vi "Configure Timing.vi"(8 "error in":errorcluster, 11 "DAQmx Base Configure Strategy in":refnum<class "DAQmx Base Configure Strategy.lvclass">) -> (0 "error out":errorcluster, 3 "DAQmx Base Configure Strategy out":refnum<class "DAQmx Base Configure Strategy.lvclass">)   [LabVIEW 2024, in "DAQmx Base Configure Strategy.lvclass"]
uses:
  DAQmx Base Configure Strategy.lvclass
  DAQmx Base Configure Strategy.lvclass/DAQmx Base Configure Strategy.ctl
  65035ada-ba25-4b4b-831a-509cfaf4f843.vi
  Source/Interfaces/IConfiguration/IConfiguration.lvclass
  <vilib>/DAQmx/configure/timing.llb/DAQmx Timing (Sample Clock).vi
  <vilib>/DAQmx/configure/timing.llb/DAQmx Timing (Implicit).vi
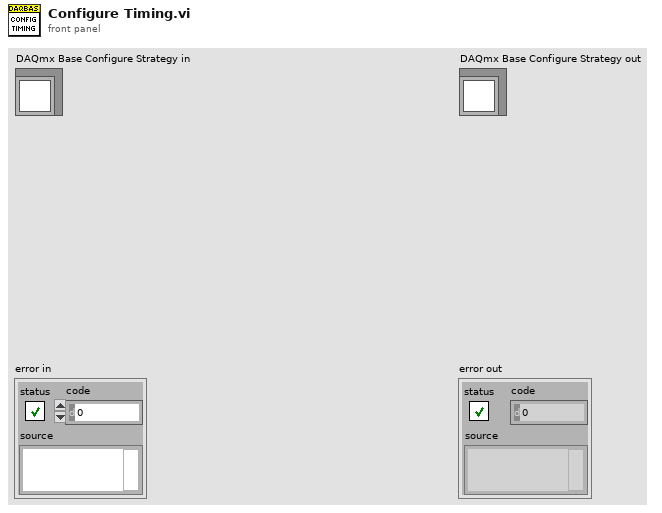
[diagram p1: front panel]
types:
  T1 = cluster{"Type":string, "SamplesPerChannel":i32, "SampleMode":string, "SampleRate":dbl, "SampleClockSource":string, "ActiveEdge":string}
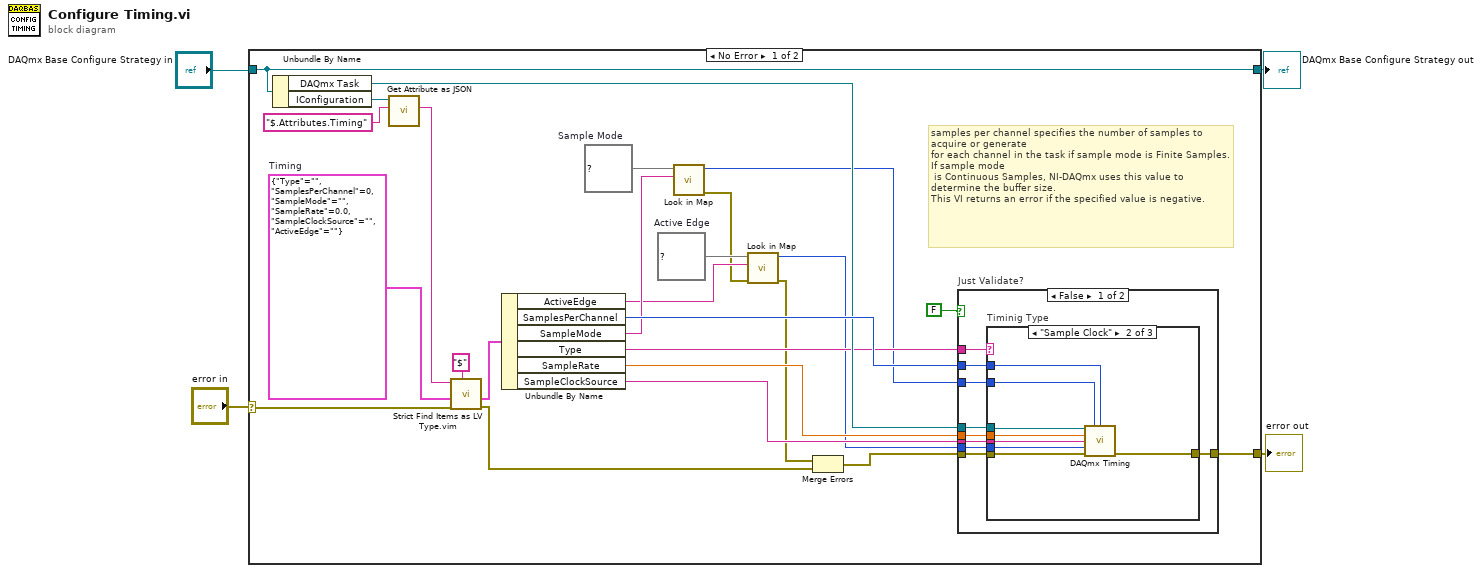
[diagram p0: block diagram]
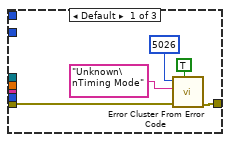
[diagram p2: hidden frame]
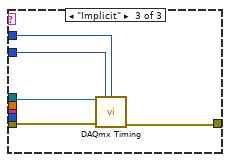
[diagram p3: hidden frame]
diagram:
  n1 = case shown="No Error" "error in" {
    selector: "error in" -> [w20 w59]
    tunnel: [w23 w59] -> w1
    tunnel: "DAQmx Base Configure Strategy in" -> [w13 w58]
    tunnel: [w13 w58] -> w3
    frame No Error {
      w16 = map{string, i32} {"Falling"=10171, "Rising"=10280}  # Active Edge
      w19 = map{string, i32} {"Continuous Samples"=10123, "Finite Samples"=10178, "Hardware Timed Single Point"=12522}  # Sample Mode
      w29 = T1 {"Type"="", "SamplesPerChannel"=0, "SampleMode"="", "SampleRate"=0.0, "SampleClockSource"="", "ActiveEdge"=""}  # Timing
      # "samples per channel specifies the number of samples to acquire or generate\nfor each channel in the task if sample mode is Finite Samples. If sample mode\n is Continuous Samples, NI-DAQmx uses this value to determine the buffer size.\nThis VI returns an error if the specified value is negative."
      n2 = Unbundle By Name(w13) -> ("DAQmx Task"=w24:refnum<k21>, "IConfiguration"=w8:refnum<class "IConfiguration.lvclass">)
      n3 = call-dynamic "Get Attribute as JSON.vi"("Attribute"="$.Attributes.Timing", "IConfiguration in"=w8) -> ("<JSON>"=w11:string)  [unwired: 7 in, 2 out]
      n4 = call "Strict Find Items as LV Type.vim"("$Path or Item Name"="$", "error in"=w20, "Data Type and Default Value"=w29, "<JSON>"=w11) -> ("error out"=w5:errorcluster, "Data out"=w28:T1)  [unwired: 5 in, 1 out]
      n5 = Unbundle By Name(w28) -> ("ActiveEdge"=w15:string, "SamplesPerChannel"=w25:i32, "SampleMode"=w18:string, "Type"=w22:string, "SampleRate"=w26:dbl, "SampleClockSource"=w27:string)
      n6 = call "Look in Map.vi"("key"=w18, "map"=w19) -> ("error out"=w7:errorcluster, "value"=w17:i32)  [unwired: 8 in]
      n7 = call "Look in Map.vi"("error in"=w7, "key"=w15, "map"=w16) -> ("error out"=w6:errorcluster, "value"=w14:i32)  [unwired: 7 in]
      n8 = Merge Errors(w6, w5) -> (w21:errorcluster)
      n9 = case "Just Validate?" shown="False" FALSE {
        tunnel: w21 -> [w38 w57]
        tunnel: w27 -> [w37 _]
        tunnel: w26 -> [w36 _]
        tunnel: w17 -> [w35 _]
        tunnel: w25 -> [w34 _]
        tunnel: w24 -> [w33 _]
        tunnel: w14 -> [w32 _]
        tunnel: [w31 w57] -> w23
        tunnel: w22 -> [w30 _]
        frame False {
          n10 = case "Timinig Type" shown="\"Sample Clock\"" w30 {
            tunnel: w38 -> [w42 w51 w54]
            tunnel: w37 -> [_ w50 _]
            tunnel: w36 -> [_ w49 _]
            tunnel: w35 -> [_ w48 w53]
            tunnel: w34 -> [_ w47 w52]
            tunnel: w33 -> [_ w46 w55]
            tunnel: [w43 w45 w56] -> w31
            tunnel: w32 -> [_ w44 _]
            frame Default {
              n11 = call <vilib>:"Error Cluster From Error Code.vi"("show call chain? (False)"=TRUE, "error in (no error)"=w42, "error message (\"\")"="Unknown\nTiming Mode" ("error message (\"\")"), "error code (0)"=5026) -> ("error out"=w43:errorcluster)  [unwired: 5 in]
            }
            frame "Sample Clock" {
              n12 = call-poly <vilib>:"DAQmx Timing.vi"("task/channels in"=w46, "sample mode"=w48, "samples per channel"=w47, "rate"=w49, "source"=w50, "active edge"=w44, "error in"=w51) -> ("error out"=w45:errorcluster)  [unwired: 7 in, 1 out]
            }
            frame "Implicit" {
              n13 = call-poly <vilib>:"DAQmx Timing.vi"("task/channels in"=w55, "sample mode"=w53, "samples per channel"=w52, "error in"=w54) -> ("error out"=w56:errorcluster)  [unwired: 10 in, 1 out]
            }
          }
        }
        frame True {
        }
      }
    }
    frame Error {
    }
  }
  "error out" <- w1
  "DAQmx Base Configure Strategy out" <- w3
